vi "RM.getAllDeviceReservationDBs.vi"(8 "error in":errorcluster, 11 "Item Ref in":T1 format="%.0x") -> (0 "error out":errorcluster, 1 "reservation dbs":variant[](array[variant]), 2 "device names":string[](array[string]), 3 "Item Ref out":T1 format="%.0x")   [LabVIEW 2016, in "FPGA Addon Shared.lvlib"]
uses:
  FPGA Addon Shared.lvlib
  <vilib>/NI Veristand/Custom Device API/Custom Device Item Ref.ctl
  <vilib>/NI Veristand/Custom Device API/Get Item Property (Variant).vi
  <vilib>/NI VeriStand/Custom Device API/Custom Device API.lvlib
  <vilib>/NI VeriStand/Custom Device Tools/Custom Device Utility Library/Custom Device Utility Library.lvlib
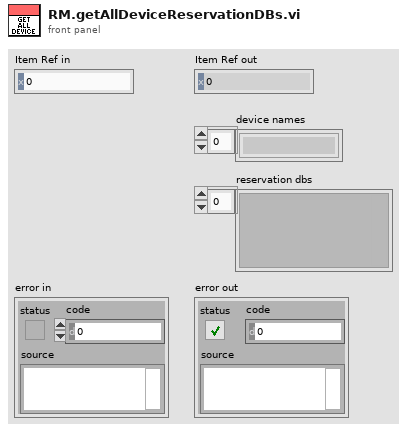
[diagram p1: front panel]
types:
  T1 = typedef "Custom Device API.lvlib/Custom Device Item Ref.ctl" = u64
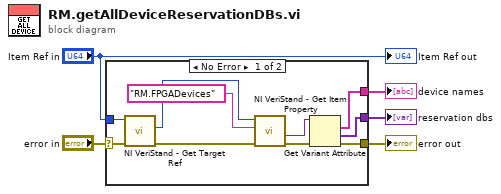
[diagram p0: block diagram]
diagram:
  n1 = case shown="No Error" "error in" {
    selector: "error in" -> [w9 w16]
    tunnel: "Item Ref in" -> [w15 _]
    tunnel: [w11 _] -> w2
    tunnel: [w10 _] -> w1
    tunnel: [w6 w16] -> w4
    frame No Error {
      n2 = call <vilib>:"NI VeriStand - Get Target Ref.vi"("error in"=w9, "Item Ref in"=w15) -> ("error out"=w8:errorcluster, "Target Ref"=w14:T1)  [unwired: 6 in, 2 out]
      n3 = call-poly <vilib>:"NI VeriStand - Get Item Property.vi"("error in (no error)"=w8, "Property Name"="RM.FPGADevices", "Item Ref in"=w14) -> ("error out"=w7:errorcluster, "Value"=w12:variant)  [unwired: 5 in, 2 out]
      n4 = Get Variant Attribute(Variant=w12, error in=w7) -> (names=w10:string[], values=w11:variant[], error out=w6:errorcluster)  [unwired: 2 in, 1 out]
    }
    frame Error {
    }
  }
  "error out" <- w4
  "reservation dbs" <- w2
  "device names" <- w1
  "Item Ref out" <- "Item Ref in"
